vi "Command Finished.vi"(8 "error in (no error)":errorcluster, 11 "Command in":refnum<class "Command.lvclass">) -> (0 "error out":errorcluster, 3 "Command out":refnum<class "Command.lvclass">)   [LabVIEW 2013]
uses:
  Command.lvclass
  <vilib>/ActorFramework/Actor/Actor.lvclass
  Command Processor/Command Processor Messages/Command Finished Msg/Command Finished Msg.lvclass
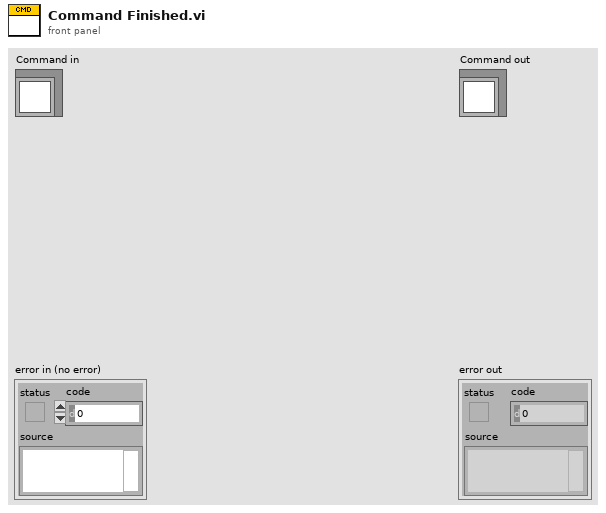
[diagram p1: front panel]
types:
  T1 = typedef "Robot Actors.lvlib/Command.lvlib/Command.lvclass/Command Status.ctl" = cluster{"Command Name":string, "Command Start Time":timestamp, "Command End Time":timestamp, "Is Command Finished?":bool, "Command ID":dbl, "Command State":T2}
  T2 = typedef "Robot Actors.lvlib/Command.lvlib/Command.lvclass/Command States.ctl" = enum16{"Unknown", "Started", "Stopped", "Finished"}
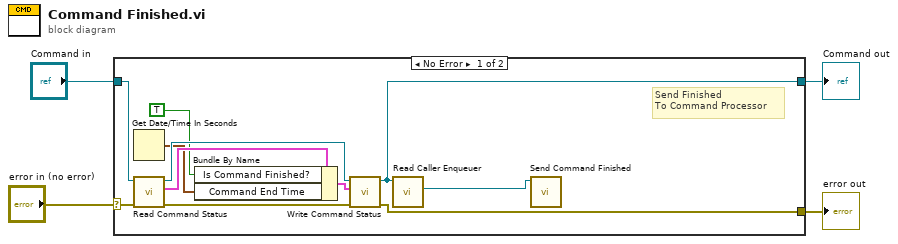
[diagram p0: block diagram]
diagram:
  n1 = case shown="No Error" "error in (no error)" {
    selector: "error in (no error)" -> [w8 w17]
    tunnel: [w6 w17] -> w3
    tunnel: [w9 w16] -> w1
    tunnel: "Command in" -> [w14 w16]
    frame No Error {
      # "Send Finished\nTo Command Processor"
      n2 = Get Date/Time In Seconds() -> (seconds since 1Jan1904=w10:timestamp)
      n3 = call-dynamic "Read Command Status.vi"("error in (no error)"=w8, "Command in"=w14) -> ("error out"=w7:errorcluster, "Command Status"=w13:T1, "Command out"=w15:refnum<class "Command.lvclass">)  [unwired: 7 in]
      n4 = Bundle By Name(cluster=w13, "Is Command Finished?"=TRUE, "Command End Time"=w10) -> (w12:T1)
      n5 = call-dynamic "Write Command Status.vi"("error in (no error)"=w7, "Command Status"=w12, "Command in"=w15) -> ("error out"=w6:errorcluster, "Command out"=w9:refnum<class "Command.lvclass">)  [unwired: 7 in]
      n6 = call <vilib>:"Read Caller Enqueuer.vi"("Actor"=w9) -> ("Caller Enqueuer"=w5:refnum<class "Message Enqueuer.lvclass">)  [unwired: 10 in]
      n7 = call "Send Command Finished.vi"("Message Enqueuer"=w5) -> ()  [unwired: 9 in, 2 out]
    }
    frame Error {
    }
  }
  "error out" <- w3
  "Command out" <- w1
